vi "Ton.vi"(5 "Ton":dbl=1000.0, 7 "input":bool, 11 "error in":errorcluster) -> (4 "elapsed time (ms)":i32, 6 "Pulse":bool, 8 "on":i32, 10 "Binary out":bool, 15 "error out":errorcluster)   [LabVIEW 2022 SP3]
uses:
  <vilib>/functionblocks/FB Core/FB Core.xnode
  <vilib>/functionblocks/Counter/Pulse Timer/Pulse Timer.vi
  <vilib>/functionblocks/NI_FunctionBlock Libraries.lvlib
  <vilib>/functionblocks/Counter/Timer Off Delay/Timer Off Delay.vi
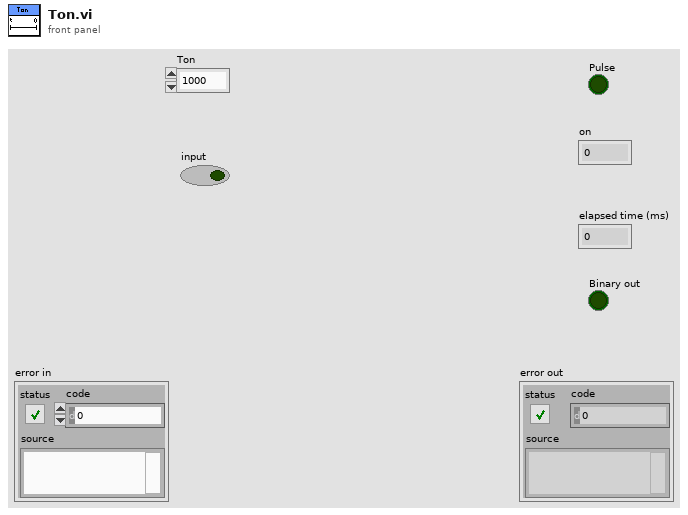
[diagram p1: front panel]
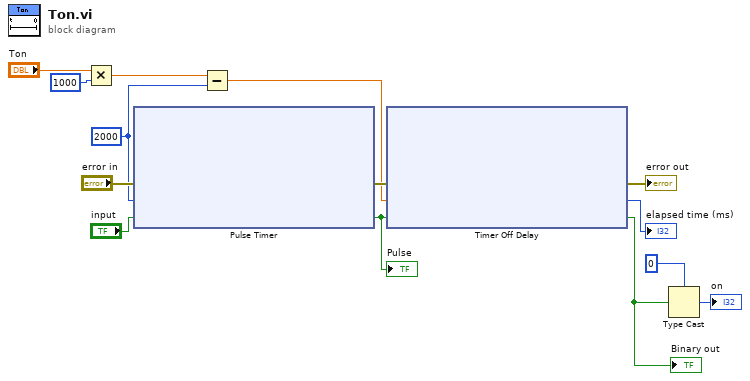
[diagram p0: block diagram]
diagram:
  w2 = 2000 ("preset time (ms)")
  n1 = Multiply(x="Ton", y=1000) -> (x*y=w3:dbl)
  n2 = xnode "Pulse Timer"("error in"="error in", "preset time (ms)"=w2, "input"="input") -> ("error out"=w8:errorcluster, "output"=w7:bool)  [unwired: 1 out]
  "Pulse" <- w7
  n3 = Subtract(x=w3, y=w2) -> (x-y=w1:dbl)
  n4 = xnode "Timer Off Delay"("error in"=w8, "preset time (ms)"=w1, "input"=w7) -> ("error out"=→"error out":errorcluster, "elapsed time (ms)"=→"elapsed time (ms)":i32, "output"=w5:bool)
  "Binary out" <- w5
  n5 = Type Cast(type=0, x=w5) -> (*(type *) &x=→"on":i32)
